vi "Read Context.vi"(8 "error in":errorcluster, 11 "State in":refnum<class "State Pattern.lvclass">) -> (0 "error out":errorcluster, 2 "Context":refnum<class "State Pattern.lvclass">, 3 "State out":refnum<class "State Pattern.lvclass">)   [LabVIEW 2021, in "State Pattern.lvclass"]
uses:
  State Pattern.lvclass
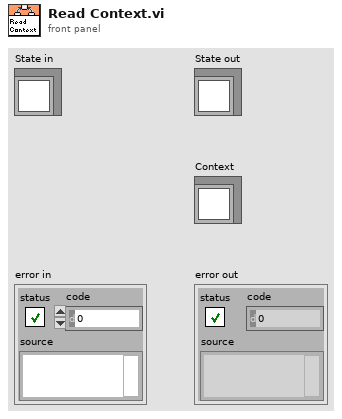
[diagram p1: front panel]
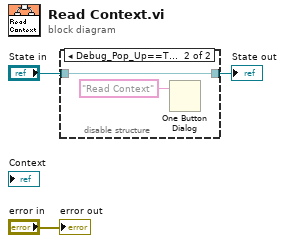
[diagram p0: block diagram]
diagram:
  n1 = disable-structure shown="Debug_Pop_Up==TRUE" {
    disable-tunnel: [w4 w5] -> w2
    disable-tunnel: "State in" -> [w4 w5]
    frame condition #0 (active) {
    }
    frame condition #1 {
      n2 = One Button Dialog(message="Read Context") -> ()  [unwired: 1 in, 1 out]
    }
  }
  "State out" <- w2
  "error out" <- "error in"
